vi "GenErrorParse.vi"(11 "register values":u16[](array[numeric]) format="%b") -> (1 "Warning":bool, 2 "SystemFault":bool, 3 "Alarms":string[](array[string]))   [LabVIEW 2014]
panel:
  # "0 0 0 1 1 1 1 1 0 0 1 0 0 0 1 1"
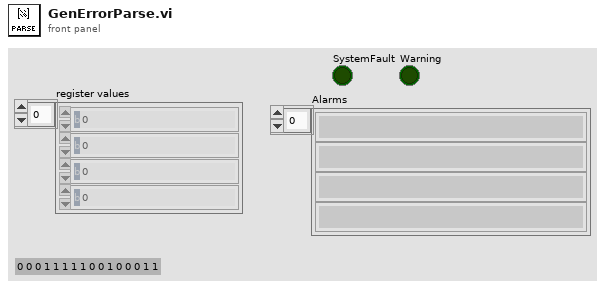
[diagram p1: front panel]
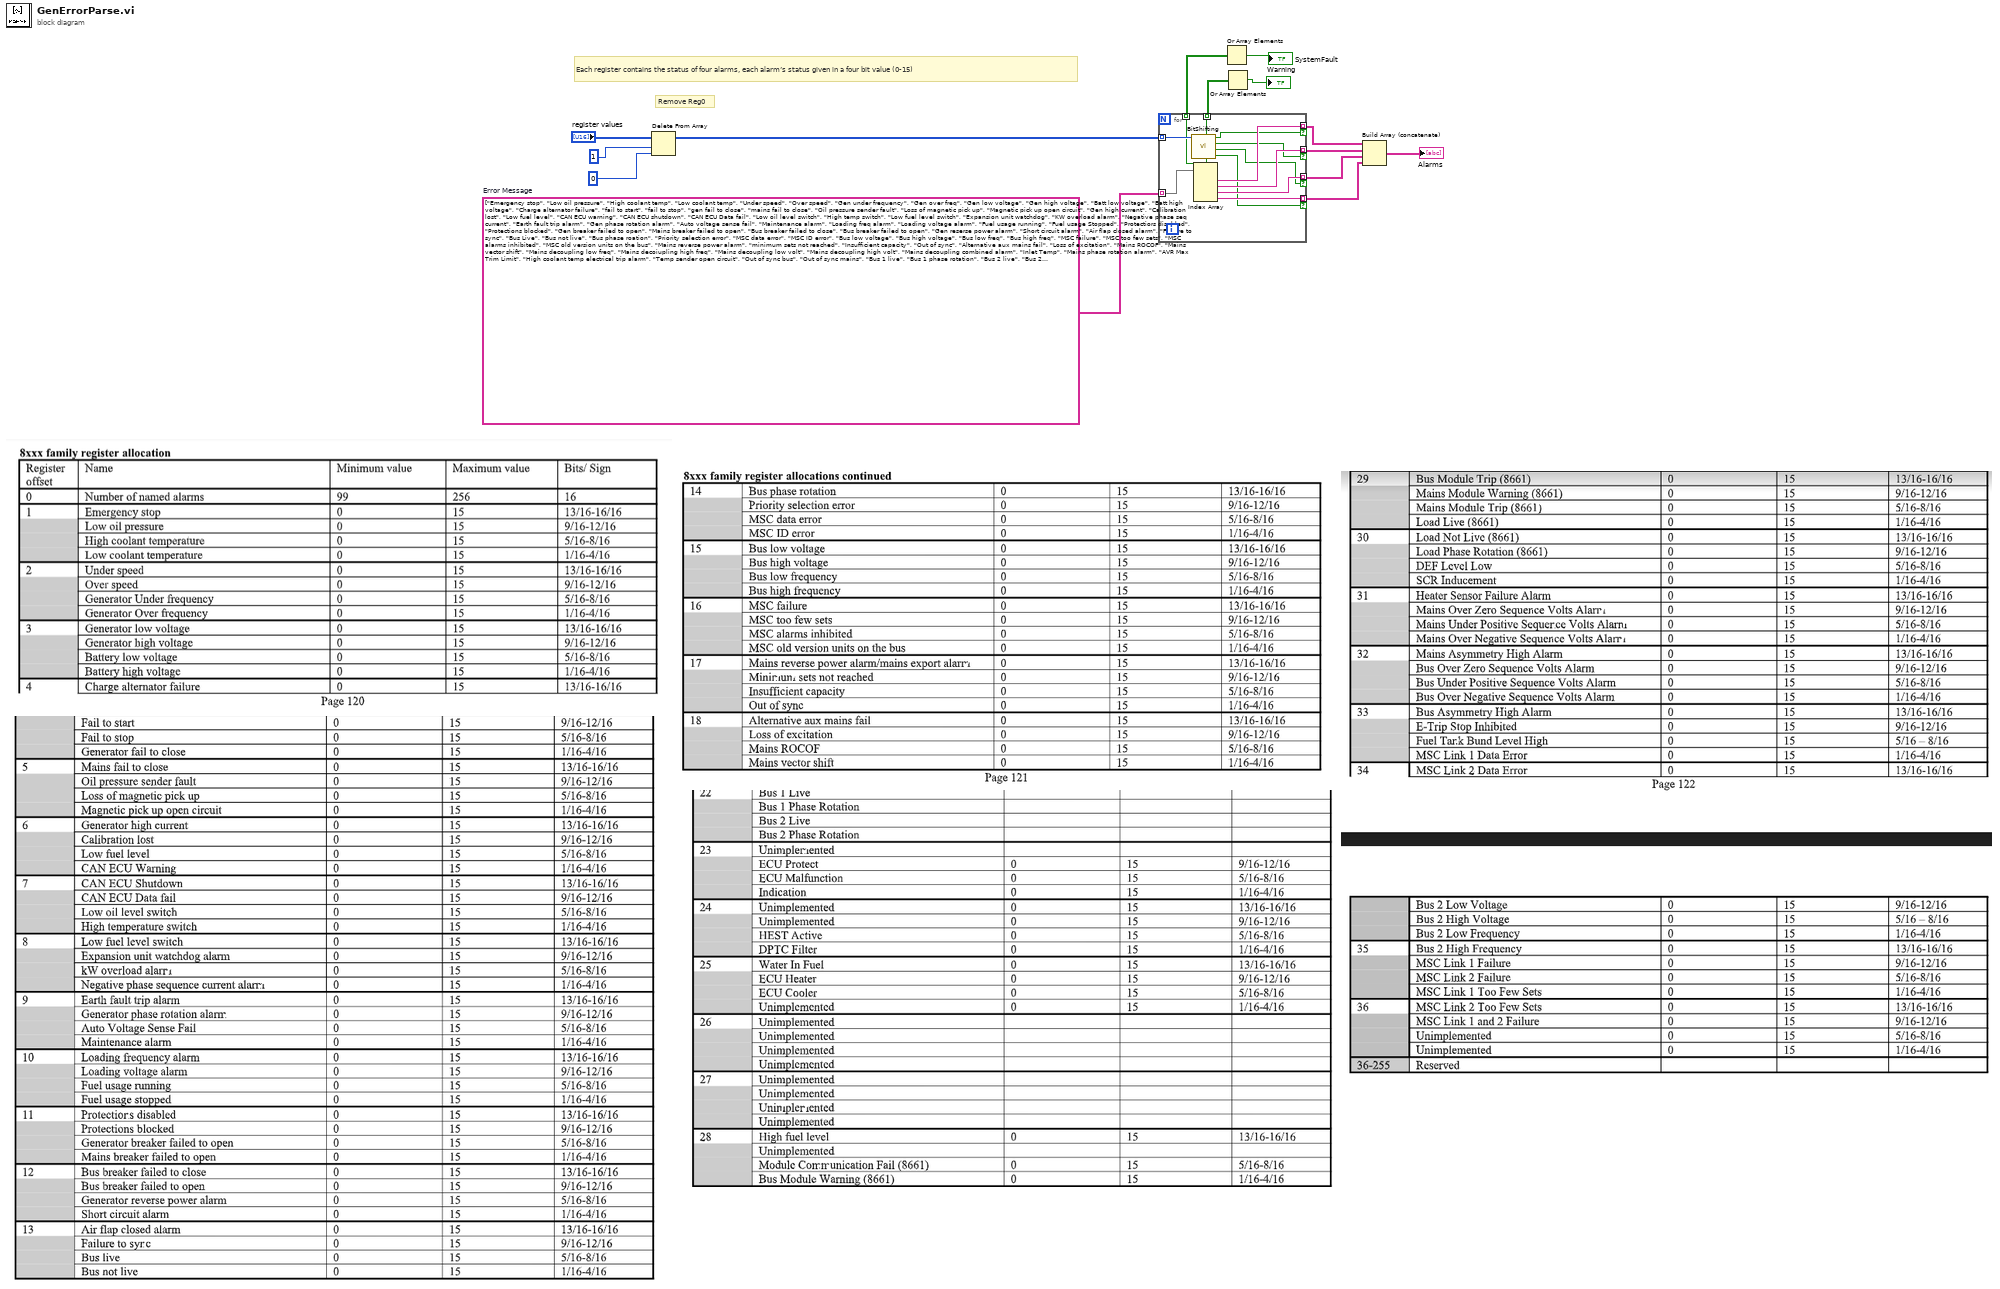
[diagram p0: block diagram]
diagram:
  w10 = string[][] [["Emergency stop", "Low oil pressure", "High coolant temp", "Low coolant temp"], ["Under speed", "Over speed", "Gen under frequency", "Gen over freq"], ["Gen low voltage", "Gen high voltage", "Batt low voltage", "Batt high voltage"], ["Charge alternator failure", "fail to start", "fail to stop", "gen fail to close"], ["mains fail to close", "Oil pressure sender fault", "Loss of magnetic pick up", "Magnetic pick up open circuit"], ["Gen high current", "Calibration lost", "Low fuel level", "CAN ECU warning"], ["CAN ECU shutdown", "CAN ECU Data fail", "Low oil level switch", "High temp switch"], ["Low fuel level switch", "Expansion unit watchdog", "KW overload alarm", "Negative phase seq current"], ["Earth fault trip alarm", "Gen phase rotation alarm", "Auto voltage sense fail", "Maintenance alarm"], ["Loading freq alarm", "Loading voltage alarm", "Fuel usage running", "Fuel usage Stopped"], ["Protectiors disabled", "Protections blocked", "Gen breaker failed to open", "Mains breaker failed to open"], ["Bus breaker failed to close", "Bus breaker failed to open", "Gen reserse power alarm", "Short circuit alarm"], ["Air flap closed alarm", "Failure to sync", "Bus Live", "Bus not live"], ["Bus phase roation", "Priority selection error", "MSC data error", "MSC ID error"], ["Bus low voltage", "Bus high voltage", "Bus low freq", "Bus high freq"], ["MSC failure", "MSC too few sets", "MSC alarms inhibited", "MSC old version units on the bus"], ["Mains reverse power alarm", "minimum sets not reached", "Insufficient capacity", "Out of sync"], ["Alternative aux mains fail", "Loss of excitation", "Mains ROCOF", "Mains vector shift"], ["Mains decoupling low freq", "Mains decoiupling high freq", "Mains decoupling low volt", "Mains decoupling high volt"], ["Mains decoupling combined alarm", "Inlet Temp", "Mains phase rotation alarm", "AVR Max Trim Limit"], ["High coolant temp electrical trip alarm", "Temp sender open circuit", "Out of sync bus", "Out of sync mains"], ["Bus 1 live", "Bus 1 phase rotation", "Bus 2 live", "Bus 2 phase rotation"], ["Unimplemented", "ECU protect", "ECU Malfunction", "Indication"], ["Unimplemented", "Unimplemented", "HEST active", "DPTC filter"], ["Water in fuel", "ECU heater", "ECU cooler", "Unimplemented"], ["Unimplemented", "Unimplemented", "Unimplemented", "Unimplemented"], ["Unimplemented", "Unimplemented", "Unimplemented", "Unimplemented"], ["High fuel level", "Unimplemented", "Module Com Fail (8661)", "Bus module Warning (8661)"], ["Bus module trip (8661)", "Mains module warning (8661)", "Mains module trip (8661)", "Load Live (8661)"], ["Load not Live (8661)", "Load Phase Rotation (8661)", "DEF level low", "SCR inducement"], ["Heater sensor failure alarm", "Mains over zero seq volts", "Main under positive seq volts", "Mains over negative seq volts"], ["Mains asymmetry high alarm", "Bus over zero seq volts alarm", "Bus under positive seq volts alarm", "Bus over negative seq volts alarm"], ["Bus Asymmetry high alarm", "E-Trip stop inhibited", "Fuel tank bund level high", "MSC link 1 data error"], ["MSC link 2 data error", "Bus 2 low volt", "Bus 2 high volt", "Bus 2 low freq"], ["Bus 2 high freq", "MSC Link 1 Failure", "MSC Link 2 Failure", "MSC Link 1 too few sets"], ["MSC Link 2 too few sets", "MSC Link 1 and 2 failure", "Unimplemented", "Unimplemented"]]  # Error Message
  # "Each register contains the status of four alarms, each alarm’s status given in a four bit value (0-15)"
  # "Remove Reg0"
  n1 = Delete From Array(array="register values", length=1, index=0) -> (array with subset deleted=w11:u16[])  [unwired: 1 out]
  n2 = for {
    tunnel: w11 -> [w26] mode=indexing
    tunnel: w10 -> [w25] mode=indexing
    tunnel: [w24] -> w9 mode=indexing if=w20
    tunnel: [w23] -> w8 mode=indexing if=w19
    tunnel: [w22] -> w7 mode=indexing if=w18
    tunnel: [w21] -> w6 mode=indexing if=w17
    tunnel: [w16] -> w4 mode=indexing
    tunnel: [w15] -> w3 mode=indexing
    n3 = call "BitShifting.vi"("register in"=w26) -> ("4-1 Error"=w17:bool, "8-5 Error"=w18:bool, "12-9 Error"=w19:bool, "16-13 Error"=w20:bool, "SystemFault"=w15:bool, "Warning"=w16:bool)  [unwired: 5 in]
    n4 = Index Array(array=w25) -> (element #1=w24:string, element #2=w23:string, element #3=w22:string, element #4=w21:string)  [unwired: 4 in]
  }
  n5 = Or Array Elements(Boolean array=w3) -> (logical OR=→"SystemFault":bool)
  n6 = Or Array Elements(Boolean array=w4) -> (logical OR=→"Warning":bool)
  n7 = Build Array (concatenate)(w9, w8, w7, w6) -> (→"Alarms":string[])
